vi "XNET UDP Socket Read (Binary).vi"(8 "error in":errorcluster, 9 "timeout ms (25000)":i32=25000, 10 "max size (548)":i32=548, 11 "socket in":refnum<k20>) -> (0 "error out":errorcluster, 2 "data":u8[](array[numeric]), 3 "socket out":refnum<k20>, 4 "remote port":u16, 6 "remote address":string)   [LabVIEW 2018]
doc: "Reads a binary datagram from a UDP socket."
uses:
  nixlvapi.dll
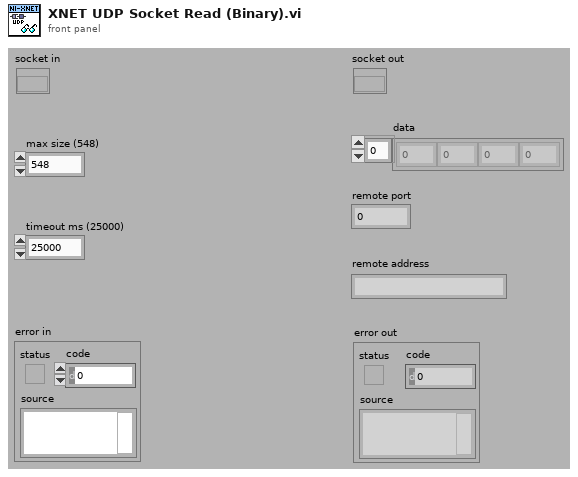
[diagram p1: front panel]
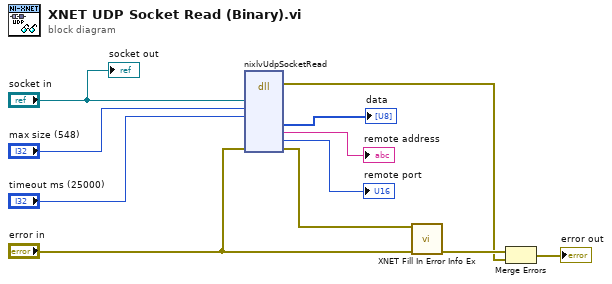
[diagram p0: block diagram]
diagram:
  n1 = dll-call lib="nixlvapi.*" fn="nixlvUdpSocketRead" label="Call Library"("socketRef"="socket in", "bytesToRead"="max size (548)", "timeoutMs"="timeout ms (25000)", "errorInOut"="error in") -> (error out=w9:errorcluster, "lvData"=→"data":u8[], "remoteAddress"=→"remote address":string, "remotePort"=→"remote port":u16, "errorInOut"=w11:errorcluster)  [unwired: 3 in, 8 out]
  n2 = call "XNET Fill In Error Info Ex.vi"("error xnet"=w11, "error in"="error in") -> ("error out"=w10:errorcluster)  [unwired: 13 in]
  n3 = Merge Errors(w10, w9) -> (→"error out":errorcluster)
  "socket out" <- "socket in"
